vi "Read waveform.vi"(4 "Channel":string="wave", 6 "Note":string="Блок формирования кадра", 8 "error in (no error)":errorcluster) -> (0 "error out":errorcluster, 2 "waveform out":waveform(dbl))   [LabVIEW 2019]
uses:
  <vilib>/addons/_NIFileIO/SV TDMS Read Waveform (1 Ch).vi
  <vilib>/Utility/config.llb/Read Key (Double).vi
  <vilib>/Utility/config.llb/NI_LVConfig.lvlib
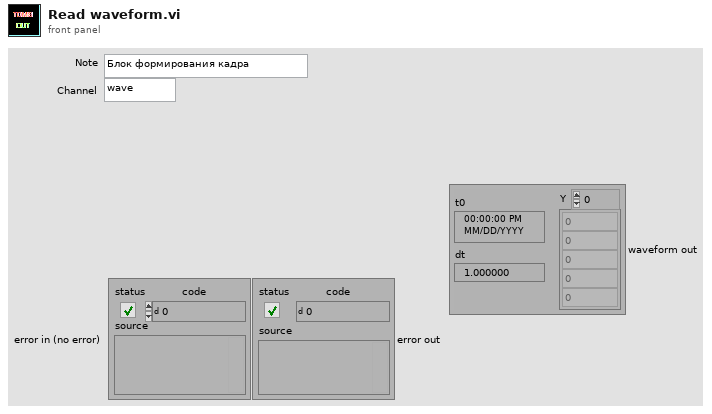
[diagram p1: front panel]
types:
  T1 = enum16{"open", "open or create", "create or replace", "create", "open (read-only)"}
  T2 = typedef "NI_LVConfig.lvlib/Config Data RefNum.ctl" = refnum<k1>
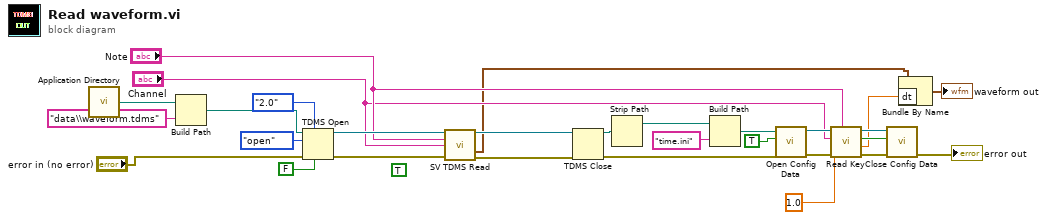
[diagram p0: block diagram]
diagram:
  (unwired) TRUE ("eof")
  n1 = call <vilib>:"Application Directory.vi"() -> ("Application Directory"=w28:path)
  n2 = Build Path(base path=w28, name or relative path="data\\waveform.tdms") -> (appended path=w26:path)
  n3 = TDMS Open(6:FALSE ("disable buffering? (T)"), 7:enum16{"1.0", "2.0"}."2.0" ("file format version (2.0)"), 8:"error in (no error)", 10:T1."open" ("operation (0:open)"), 11:w26) -> (0:w20:errorcluster, 3:w22:refnum<k34>)  [unwired: 2 in]
  n4 = call-poly <vilib>:"SV TDMS Read.vi"("tdms file"=w22, "group name in"="Note", "channel name in"="Channel", "error in"=w20) -> ("tdms file out"=w21:refnum<k34>, "waveform"=w2:waveform(dbl), "error out"=w19:errorcluster)  [unwired: 6 in, 3 out]
  n5 = TDMS Close(8:w19, 11:w21) -> (0:w13:errorcluster, 3:w16:path)
  n6 = Strip Path(path=w16) -> (stripped path=w18:path)  [unwired: 1 out]
  n7 = Build Path(base path=w18, name or relative path="time.ini") -> (appended path=w15:path)
  n8 = call <vilib>:"Open Config Data.vi"("error in (no error)"=w13, "create file if necessary (T)"=TRUE, "configuration file path"=w15) -> ("error out"=w8:errorcluster, "refnum"=w9:T2)  [unwired: 6 in, 1 out]
  n9 = call-poly <vilib>:"Read Key.vi"("section"="Note", "error in (no error)"=w8, "default value"=1.0, "key"="Channel", "refnum"=w9) -> ("error out"=w12:errorcluster, "value"=w3:dbl, "found?"=w11:bool, "refnum out"=w10:T2)  [unwired: 3 in]
  n10 = call <vilib>:"Close Config Data.vi"("error in (no error)"=w12, "write file if changed (T)"=w11, "refnum"=w10) -> ("error out"=→"error out":errorcluster)  [unwired: 7 in, 1 out]
  n11 = Bundle By Name(cluster=w2, "dt"=w3) -> (→"waveform out":waveform(dbl))
